vi "Quick Read.vi"(8 "error in (no error)":errorcluster, 11 "Fluke Multimeter.lvclass In":refnum<class "Fluke Multimeter.lvclass">) -> (0 "error out":errorcluster, 1 "unit":string, 2 "measurement":dbl format="%^.6e", 3 "Fluke Multimeter.lvclass Out":refnum<class "Fluke Multimeter.lvclass">)   [LabVIEW 2017, in "Fluke Multimeter.lvclass"]
doc: "Performs a quick read. Must use Init & Config Method before use."
uses:
  Fluke Multimeter.lvclass
  Fluke Multimeter.lvclass/Fluke Multimeter.ctl
  Fluke 8840/Fluke 8840.lvlib
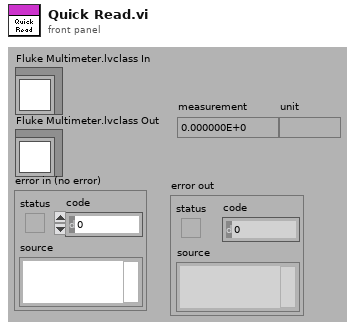
[diagram p1: front panel]
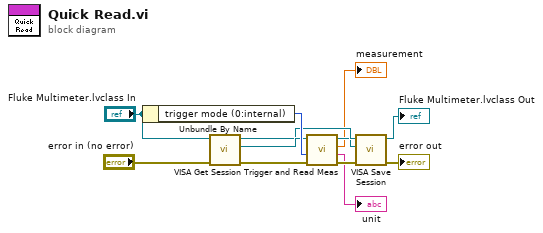
[diagram p0: block diagram]
diagram:
  n1 = Unbundle By Name("Fluke Multimeter.lvclass In") -> ("trigger mode (0:internal)"=w9:u16)
  n2 = call-dynamic "VISA Get Session.vi"("error in (no error)"="error in (no error)", "Instrument.lvclass in"="Fluke Multimeter.lvclass In") -> ("error out"=w8:errorcluster, "VISA Resource Name"=w7:refnum<visa-resource-name>, "Instrument.lvclass out"=w6:refnum<class "Fluke Multimeter.lvclass">)  [unwired: 6 in, 1 out]
  n3 = call "Trigger and Read Meas.vi"("error in (no error)"=w8, "trigger mode (0:internal)"=w9, "VISA resource name"=w7) -> ("error out"=w4:errorcluster, "unit"=→"unit":string, "measurement"=→"measurement":dbl, "VISA resource name out"=w5:refnum<visa-resource-name>)  [unwired: 5 in]
  n4 = call-dynamic "VISA Save Session.vi"("error in (no error)"=w4, "VISA Resource Name"=w5, "Instrument.lvclass in"=w6) -> ("error out"=→"error out":errorcluster, "Instrument.lvclass out"=→"Fluke Multimeter.lvclass Out":refnum<class "Fluke Multimeter.lvclass">)  [unwired: 7 in]
